vi "Assert Wrapper.vi"(6 "error code (1)":i32=1, 7 "Message":string, 8 "error in (no error)":errorcluster, 11 "Assert?":bool) -> (0 "error out":errorcluster)   [LabVIEW 2009]
uses:
  Assert Factory Global/Assert Factory Global.lvclass
  Assert Factory/Assert Factory.lvclass
  Assert/Assert.lvclass
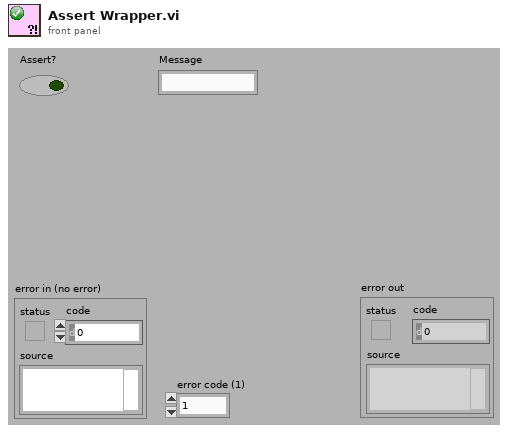
[diagram p1: front panel]
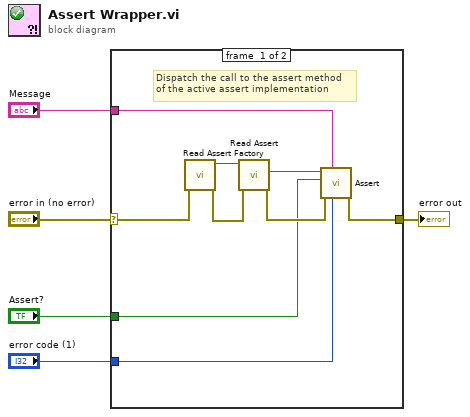
[diagram p0: block diagram]
diagram:
  n1 = case shown="No Error" "error in (no error)" {
    selector: "error in (no error)" -> [w7 w15]
    tunnel: [w11 w15] -> w5
    tunnel: "error code (1)" -> [w10 _]
    tunnel: "Message" -> [w9 _]
    tunnel: "Assert?" -> [w8 _]
    frame #0 {
      # "Dispatch the call to the assert method\nof the active assert implementation"
      n2 = call "Read Assert Factory.vi"("error in (no error)"=w7) -> ("error out"=w6:errorcluster, "Assert Factory"=w14:refnum<class "Assert Factory.lvclass">)  [unwired: 9 in]
      n3 = call-dynamic "Read Assert.vi"("error in (no error)"=w6, "Assert Factory in"=w14) -> ("error out"=w12:errorcluster, "Assert"=w13:refnum<class "Assert.lvclass">)  [unwired: 7 in, 1 out]
      n4 = call-dynamic "Assert.vi"("error code (1)"=w10, "Message"=w9, "error in (no error)"=w12, "Assert?"=w8, "Assert in"=w13) -> ("error out"=w11:errorcluster)  [unwired: 5 in, 1 out]
    }
    frame #1 {
    }
  }
  "error out" <- w5
